vi "CIC_5decimate_1cycle_for_5761.vi"(7 "reset":bool, 8 "valid in":bool, 11 "Data in":fxp<+/-,16,14>) -> (0 "valid out":bool, 3 "Data out":fxp<+/-,16,14>)   [LabVIEW 2018]
uses:
  <vilib>/rvi/IPIntegrationNode/IPINode_Typedef/niFpgaIPINodeSupportedFamilies.ctl
  <vilib>/rvi/IPIntegrationNode/IPINode_Utilities/niFpgaIPINodeSimCore.vi
  <vilib>/rvi/FXPMathLib/FxpInterpret/XNode/nifxpmath_Interpret.xnode
  <vilib>/rvi/XilinxIP/XIPIN_XNode/niFpgaXIPIN.xnode
  CIC_5decimate_1cycle_for_5761/xsim.dir/CIC_5decimate_1cycle_for_5761_978BFF4F28994E7297D8CFB5DA7FCEAF/xsimk_978BFF4F28994E7297D8CFB5DA7FCEAF.dll
  <vilib>/rvi/IPIntegrationNode/IPINode_Xnode/niFpgaIPINode.xnode
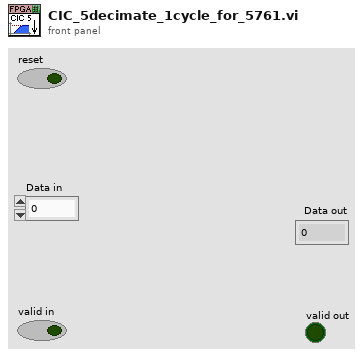
[diagram p1: front panel]
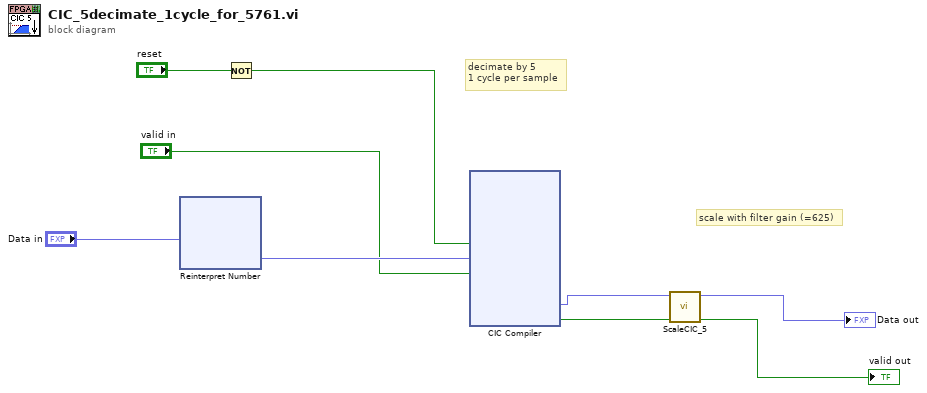
[diagram p0: block diagram]
diagram:
  # "decimate by 5\n1 cycle per sample"
  # "scale with filter gain (=625)"
  n1 = xnode "Reinterpret Number"("x"="Data in") -> ("y"=w4:fxp<+,16,16>)
  n2 = Not(x="reset") -> (.not. x?=w5:bool)
  n3 = xnode ("CIC Compiler")("aresetn"=w5, "s_axis_data_tdata"=w4, "s_axis_data_tvalid"="valid in") -> ("m_axis_data_tdata"=w2:fxp<+/-,32,32>, "m_axis_data_tvalid"=w1:bool)  [unwired: 1 in, 1 out]
  n4 = call "ScaleCIC_5.vi"("input valid"=w1, "x"=w2) -> ("valid out"=→"valid out":bool, "Data out"=→"Data out":fxp<+/-,16,14>)  [unwired: 8 in]
